vi "mdps.vi"() -> ()   [LabVIEW 2015]
uses:
  <vilib>/Utility/error.llb/DialogType.ctl
  <vilib>/DAQmx/read.llb/DAQmx Read (Digital Bool 1Line 1Point).vi
  <vilib>/DAQmx/read.llb/DAQmx Read (Analog 1D DBL NChan 1Samp).vi
  <vilib>/DAQmx/write.llb/DAQmx Write (Analog 1D DBL NChan 1Samp).vi
  <vilib>/DAQmx/write.llb/DAQmx Write (Digital Bool 1Line 1Point).vi
  <vilib>/DAQmx/write.llb/DAQmx Write (Counter Frequency 1Chan 1Samp).vi
  <vilib>/DAQmx/create/channels.llb/DAQmx Create Channel (CO-Pulse Generation-Frequency).vi
  <vilib>/DAQmx/configure/timing.llb/DAQmx Timing (Implicit).vi
  mdps_global.vi
  <vilib>/DAQmx/miscellaneous.llb/DAQmx Fill In Error Info.vi
  <vilib>/DAQmx/create/channels.llb/DAQmx Create Channel (AI-Voltage-Basic).vi
  <vilib>/DAQmx/create/channels.llb/DAQmx Create Channel (DI-Digital Input).vi
  <vilib>/DAQmx/create/channels.llb/DAQmx Create Channel (AO-Voltage-Basic).vi
  <vilib>/DAQmx/create/channels.llb/DAQmx Create Channel (DO-Digital Output).vi
  <vilib>/Utility/inputDevices.llb/mouseAcquire.vi
  <vilib>/Utility/inputDevices.llb/closeMouse.vi
  <vilib>/DAQmx/configure/timing.llb/DAQmx Timing (Sample Clock).vi
  <vilib>/DAQmx/read.llb/DAQmx Read (Analog 2D DBL NChan NSamp).vi
  <vilib>/Instr/_visa.llb/VISA Configure Serial Port (Instr).vi
panel:
  out "read buffer":string
  in  "vel":i32 min=0 max=1000 step=20
  out "count 3":i32
  out "solinit":bool
  out "count 2":i32
  out "manual":bool
  out "Waveform Chart 2":dynamicdata(graph)
  out "lastval":dbl[](array[numeric])
  out "count":i32
  in  "steering":dbl(knob) min=-0.45 max=0.45 step=0.005 scale=-0.45..0.45
  out "Waveform Chart":dynamicdata(graph)
  out "coerced(x)":dbl[](array[numeric])
  out "data 2":bool
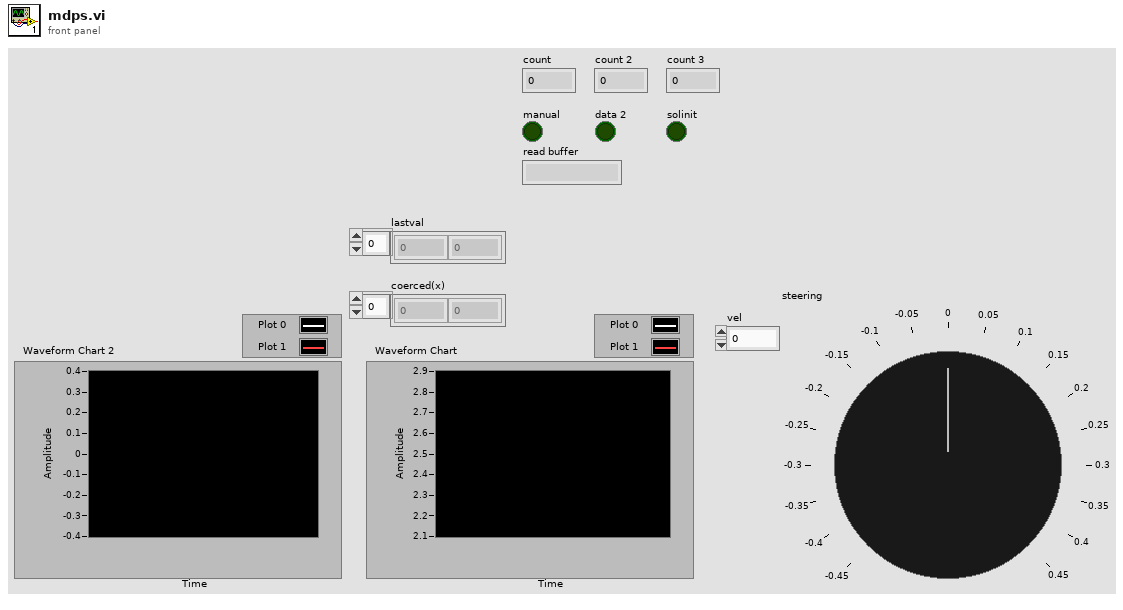
[diagram p1: front panel]
types:
  T1 = typedef "DialogType.ctl" = u16
  T2 = cluster{"button 1":bool, "button 2":bool, "button 3":bool, "button 4":bool}
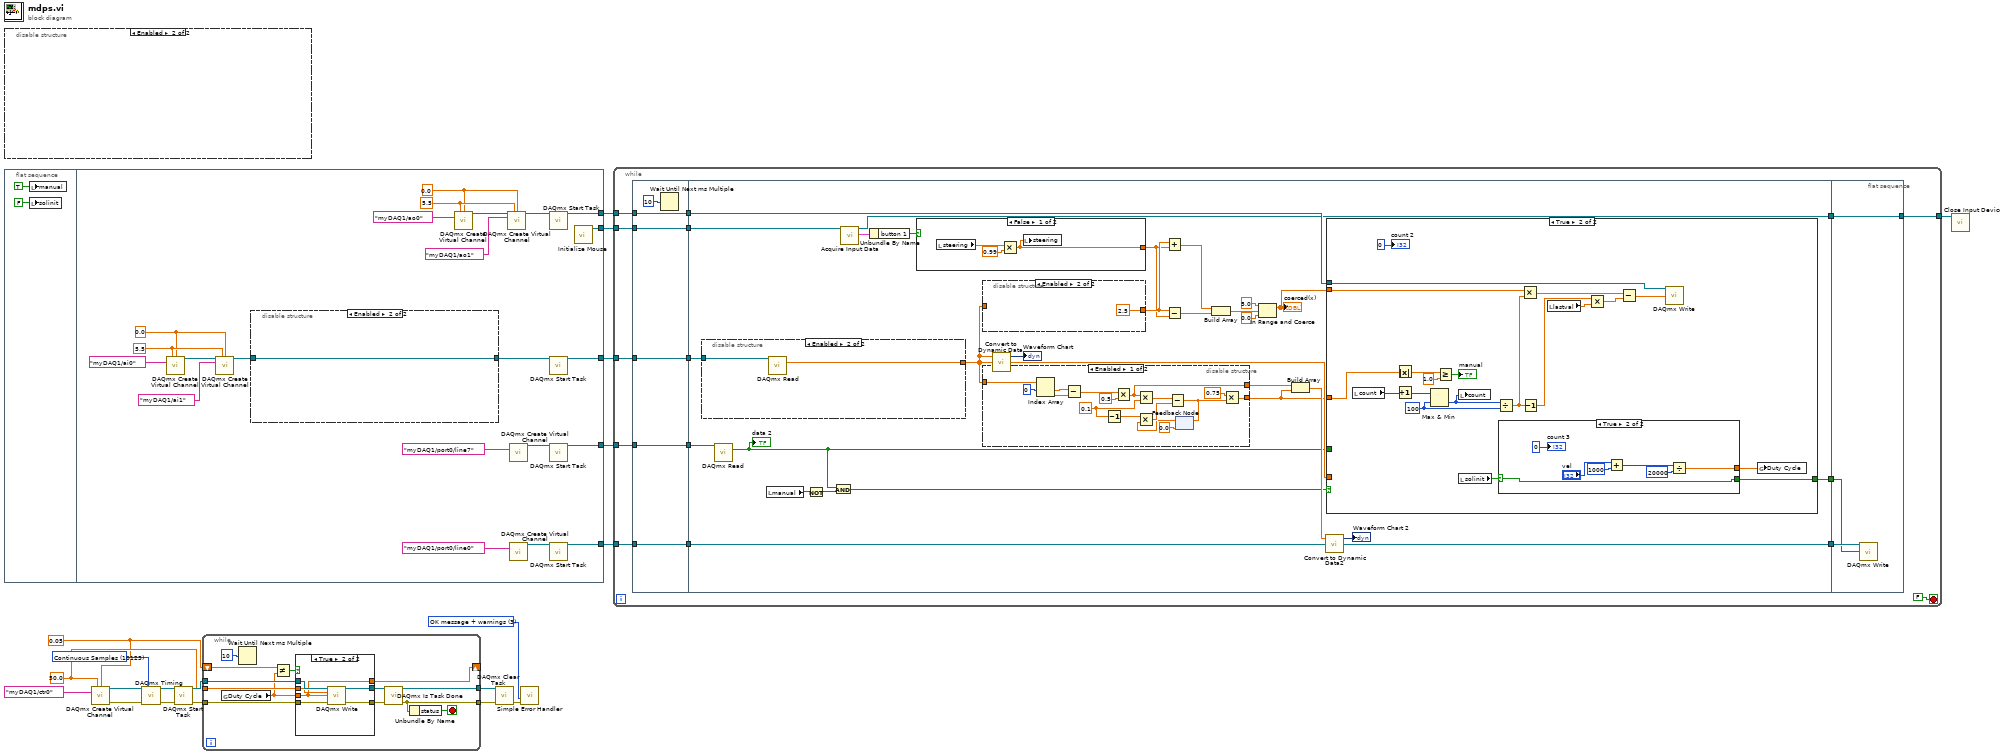
[diagram p0: block diagram]
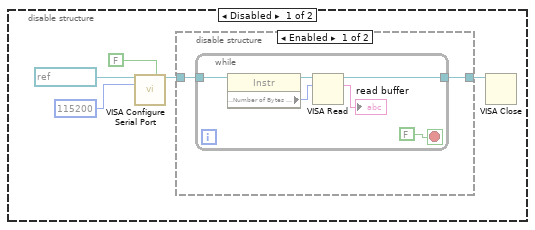
[diagram p2: hidden frame]
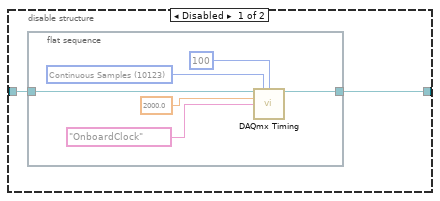
[diagram p5: hidden frame]
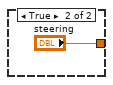
[diagram p6: hidden frame]
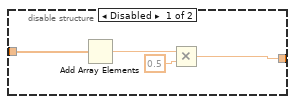
[diagram p7: hidden frame]
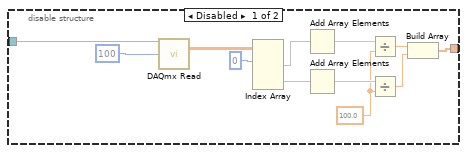
[diagram p8: hidden frame]
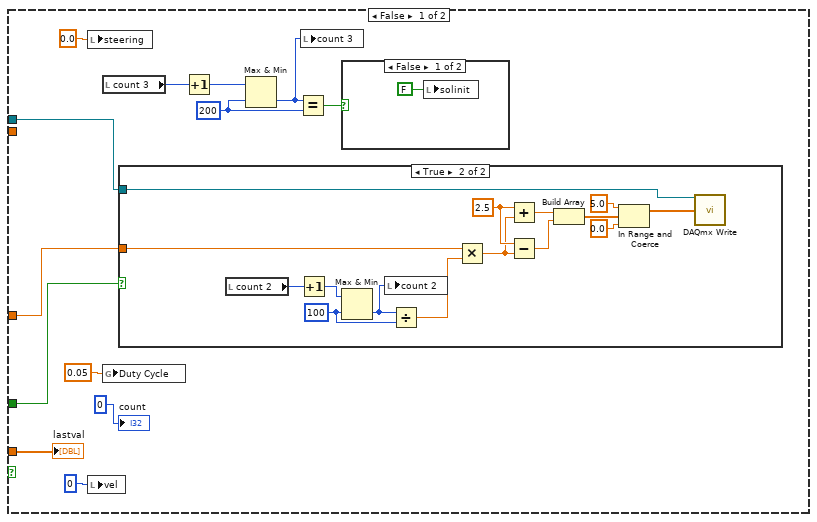
[diagram p10: hidden frame]
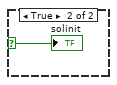
[diagram p11: hidden frame]
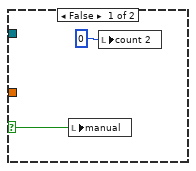
[diagram p12: hidden frame]
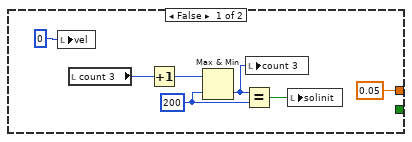
[diagram p13: hidden frame]
diagram:
  w4 = 0.05 ("Duty Cycle")
  w5 = 50.0 ("Frequency")
  w6 = T1 3 items=["no dialog", "OK message", "continue or stop message", "OK message + warnings", "continue/stop + warnings"] ("type of dialog (OK msg:1)")
  w9 = 10123 items=["Finite Samples"=10178, "Continuous Samples"=10123] ("sample mode")
  n1 = disable-structure shown="Enabled" {
    frame Disabled {
      n2 = call-poly "VISA Configure Serial Port"("VISA resource name"=refnum<visa-resource-name> "COM8", "Enable Termination\nChar (T)"=FALSE ("Enable Termination\nChar (T)"), "baud rate (9600)"=u32 115200) -> ("VISA resource name out"=w23:refnum<visa-resource-name>)  [unwired: 6 in, 6 out]
      n3 = disable-structure shown="Enabled" {
        disable-tunnel: w23 -> [w27 w34]
        disable-tunnel: [w26 w34] -> w22
        frame Enabled {
          n4 = while {
            tunnel: w27 -> [w31]
            tunnel: [w32] -> w26
            stop <- FALSE stop-if-true
            n5 = property class="Instr"(reference=w31) -> (reference out=w30:refnum<visa-resource-name>, "Serial Settings:Number of Bytes at Serial Port"=w29:u32)  [unwired: 1 in, 1 out]
            n6 = VISA Read(VISA resource name=w30, byte count=w29) -> (VISA resource name out=w32:refnum<visa-resource-name>, read buffer=→"read buffer":string)  [unwired: 1 in, 2 out]
          }
        }
        frame Disabled {
        }
      }
      n7 = VISA Close(VISA resource name=w22) -> ()  [unwired: 1 in, 1 out]
    }
    frame Enabled {
    }
  }
  n8 = flat-sequence {
    tunnel: [w53] -> w20
    tunnel: [w50] -> w19
    tunnel: [w46] -> w18
    tunnel: [w38] -> w3
    tunnel: [w37] -> w2
    frame #0 {
      n9 = local write "manual"(TRUE) -> ()
      n10 = local write "solinit"(FALSE) -> ()
    }
    frame #1 {
      w44 = 0.0 ("minimum value")
      w45 = 5.5 ("maximum value")
      w54 = 0.0 ("minimum value")
      w55 = 5.5 ("maximum value")
      n11 = call-poly <vilib>:"DAQmx Create Virtual Channel.vi"("maximum value"=w55, "minimum value"=w54, "physical channels"=tag "myDAQ1/ai0" ("Physical Channel")) -> ("task out"=w57:refnum<k21>)  [unwired: 11 in, 1 out]
      n12 = call-poly <vilib>:"DAQmx Create Virtual Channel.vi"("task in"=w57, "maximum value"=w55, "minimum value"=w54, "physical channels"=tag "myDAQ1/ai1") -> ("task out"=w43:refnum<k21>)  [unwired: 10 in, 1 out]
      n13 = disable-structure shown="Enabled" {
        disable-tunnel: w43 -> [w60 w67]
        disable-tunnel: [w59 w67] -> w42
        frame Disabled {
          n14 = flat-sequence {
            tunnel: w60 -> [w66]
            tunnel: [w65] -> w59
            frame #0 {
              w61 = 10123 items=["Finite Samples"=10178, "Continuous Samples"=10123, "Hardware Timed Single Point"=12522] ("sample mode")
              n15 = call-poly <vilib>:"DAQmx Timing.vi"("task/channels in"=w66, "sample mode"=w61, "samples per channel"=100, "rate"=2000.0, "source"=tag "OnboardClock") -> ("task out"=w65:refnum<k21>)  [unwired: 9 in, 1 out]
            }
          }
        }
        frame Enabled {
        }
      }
      n16 = call-poly <vilib>:"DAQmx Create Virtual Channel.vi"("maximum value"=w45, "minimum value"=w44, "physical channels"=tag "myDAQ1/ao0") -> ("task out"=w48:refnum<k21>)  [unwired: 11 in, 1 out]
      n17 = call-poly <vilib>:"DAQmx Create Virtual Channel.vi"("task in"=w48, "maximum value"=w45, "minimum value"=w44, "physical channels"=tag "myDAQ1/ao1") -> ("task out"=w41:refnum<k21>)  [unwired: 10 in, 1 out]
      n18 = call-poly <vilib>:"DAQmx Create Virtual Channel.vi"("lines"=tag "myDAQ1/port0/line7") -> ("task out"=w51:refnum<k21>)  [unwired: 13 in, 1 out]
      n19 = call-poly <vilib>:"DAQmx Create Virtual Channel.vi"("lines"=tag "myDAQ1/port0/line0") -> ("task out"=w40:refnum<k21>)  [unwired: 13 in, 1 out]
      n20 = call <vilib>:"DAQmx Start Task.vi"("task/channels in"=w41) -> ("task out"=w46:refnum<k21>)  [unwired: 13 in, 1 out]
      n21 = call <vilib>:"DAQmx Start Task.vi"("task/channels in"=w42) -> ("task out"=w53:refnum<k21>)  [unwired: 13 in, 1 out]
      n22 = call <vilib>:"DAQmx Start Task.vi"("task/channels in"=w51) -> ("task out"=w50:refnum<k21>)  [unwired: 13 in, 1 out]
      n23 = call <vilib>:"DAQmx Start Task.vi"("task/channels in"=w40) -> ("task out"=w38:refnum<k21>)  [unwired: 13 in, 1 out]
      n24 = call <vilib>:"Initialize Mouse.vi"() -> ("device ID"=w37:refnum<k1>)  [unwired: 10 in, 1 out]
    }
  }
  n25 = call-poly <vilib>:"DAQmx Create Virtual Channel.vi"("frequency"=w5, "duty cycle"=w4, "counter"=tag "myDAQ1/ctr0" ("Counter(s)")) -> ("task out"=w14:refnum<k21>, "error out"=w17:errorcluster)  [unwired: 11 in]
  n26 = call-poly <vilib>:"DAQmx Timing.vi"("task/channels in"=w14, "sample mode"=w9, "error in"=w17) -> ("task out"=w10:refnum<k21>, "error out"=w11:errorcluster)  [unwired: 11 in]
  n27 = call <vilib>:"DAQmx Start Task.vi"("task/channels in"=w10, "error in"=w11) -> ("task out"=w13:refnum<k21>, "error out"=w16:errorcluster)  [unwired: 12 in]
  n28 = while {
    tunnel: w16 -> [w75]
    tunnel: w13 -> [w76]
    tunnel: [w80] -> w12
    tunnel: [w79] -> w7
    tunnel: w5 -> [w74]
    shift-right: [w71] -> _
    shift-left: w4 -> [w72]
    stop <- w69 stop-if-true
    n29 = global read "mdps_global.vi" "Duty Cycle"() -> (w68:dbl)
    n30 = Wait Until Next ms Multiple(millisecond multiple=u32 10) -> ()  [unwired: 1 out]
    n31 = Not Equal?(x=w72, y=w68) -> (x != y?=w73:bool)
    n32 = case shown="True" w73 {
      tunnel: [w83 w89] -> w78
      tunnel: [w82 w88] -> w77
      tunnel: w76 -> [w83 w87]
      tunnel: w75 -> [w82 w86]
      tunnel: w74 -> [_ w85]
      tunnel: w68 -> [w81 w84]
      tunnel: [w81 w84] -> w71
      frame False {
      }
      frame True {
        n33 = call-poly <vilib>:"DAQmx Write.vi"("task/channels in"=w87, "frequency"=w85, "duty cycle"=w84, "error in"=w86) -> ("task out"=w89:refnum<k21>, "error out"=w88:errorcluster)  [unwired: 9 in, 1 out]
      }
    }
    n34 = call <vilib>:"DAQmx Is Task Done.vi"("task/channels in"=w78, "error in"=w77) -> ("task out"=w80:refnum<k21>, "error out"=w79:errorcluster)  [unwired: 11 in, 1 out]
    n35 = Unbundle By Name(w79) -> ("status"=w69:bool)
  }
  n36 = call <vilib>:"DAQmx Clear Task.vi"("task in"=w12, "error in"=w7) -> ("error out"=w15:errorcluster)  [unwired: 13 in]
  n37 = call <vilib>:"Simple Error Handler.vi"("type of dialog (OK msg:1)"=w6, "error in (no error)"=w15) -> ()  [unwired: 3 in, 5 out]
  n38 = while {
    tunnel: w20 -> [w103]
    tunnel: w19 -> [w102]
    tunnel: w18 -> [w101]
    tunnel: w3 -> [w96]
    tunnel: w2 -> [w92]
    tunnel: [w90] -> w1
    stop <- FALSE stop-if-true
    n39 = flat-sequence {
      tunnel: w101 -> [w108]
      tunnel: w102 -> [w109]
      tunnel: w103 -> [w110]
      tunnel: [w110] -> w100
      tunnel: [w109] -> w99
      tunnel: [w108] -> w98
      tunnel: w96 -> [w106]
      tunnel: [w106] -> w95
      tunnel: [w105] -> w93
      tunnel: w92 -> [w105]
      tunnel: w100 -> [w126]
      tunnel: w99 -> [w137]
      tunnel: w98 -> [w136]
      tunnel: [w116] -> w97
      tunnel: w95 -> [w115]
      tunnel: [w115] -> w94
      tunnel: w93 -> [w114]
      tunnel: [w111] -> w91
      tunnel: w97 -> [w244]
      tunnel: w94 -> [w245]
      tunnel: w91 -> [w243]
      tunnel: [w243] -> w90
      frame #0 {
        n40 = Wait Until Next ms Multiple(millisecond multiple=u32 10) -> ()  [unwired: 1 out]
      }
      frame #1 {
        n41 = disable-structure shown="Enabled" {
          disable-tunnel: [w151 w159] -> w127
          disable-tunnel: w126 -> [w149 w160]
          frame Disabled {
            w154 = 100.0 ("y")
            n42 = call-poly <vilib>:"DAQmx Read.vi"("task/channels in"=w149, "number of samples per channel"=100) -> ("data"=w148:dbl[][])  [unwired: 11 in, 2 out]
            n43 = Index Array(array=w148, index (row) #1=0 ("disabled index (col)")) -> (element #1=w158:dbl[], element #2=w157:dbl[])  [unwired: 3 in]
            n44 = Add Array Elements(numeric array=w158) -> (sum=w156:dbl)
            n45 = Add Array Elements(numeric array=w157) -> (sum=w155:dbl)
            n46 = Divide(x=w156, y=w154) -> (x/y=w153:dbl)
            n47 = Divide(x=w155, y=w154) -> (x/y=w152:dbl)
            n48 = Build Array(w153, w152) -> (w151:dbl[])
          }
          frame Enabled {
            n49 = call-poly <vilib>:"DAQmx Read.vi"("task/channels in"=w160) -> ("data"=w159:dbl[])  [unwired: 12 in, 2 out]
          }
        }
        n50 = call-poly <vilib>:"DAQmx Read.vi"("task/channels in"=w137) -> ("data"=w117:bool)  [unwired: 12 in, 2 out]
        "data 2" <- w117
        n51 = local read "manual"() -> (w120:bool)
        n52 = Not(x=w120) -> (.not. x?=w119:bool)
        n53 = And(x=w117, y=w119) -> (x .and. y?=w118:bool)
        n54 = call-poly <vilib>:"Acquire Input Data.vi"("device ID"=w114) -> ("device ID"=w111:refnum<k1>, "button info"=w112:T2)  [unwired: 15 in, 2 out]
        n55 = Unbundle By Name(w112) -> ("button 1"=w113:bool)
        n56 = case shown="False" w113 {
          tunnel: [w138 "steering"] -> w122
          frame False {
            n57 = local read "steering"() -> (w139:dbl)
            n58 = Multiply(x=w139, y=0.99) -> (x*y=w138:dbl)
            n59 = local write "steering"(w138) -> ()
          }
          frame True {
          }
        }
        n60 = disable-structure shown="Enabled" {
          disable-tunnel: [w143 2.5] -> w132
          disable-tunnel: w127 -> [w142 _]
          frame Disabled {
            n61 = Add Array Elements(numeric array=w142) -> (sum=w145:dbl)
            n62 = Multiply(x=w145, y=0.5) -> (x*y=w143:dbl)
          }
          frame Enabled {
          }
        }
        n63 = disable-structure shown="Enabled" {
          disable-tunnel: [w173 _] -> w121
          disable-tunnel: w127 -> [w170 _]
          disable-tunnel: [w161 _] -> w123
          frame Enabled {
            w168 = 0.1 ("y")
            n64 = Index Array(array=w170, index #1=0 ("index")) -> (element #1=w172:dbl, element #2=w171:dbl)  [unwired: 1 in]
            n65 = Subtract(x=w172, y=w171) -> (x-y=w175:dbl)
            n66 = Decrement(x=w168) -> (x-1=w167:dbl)
            n67 = Multiply(x=w175, y=0.5) -> (x*y=w161:dbl)
            n68 = Multiply(x=w161, y=w168) -> (x*y=w166:dbl)
            n69 = feedback #1(0.0) -> (w163:dbl)
            n70 = Multiply(x=w167, y=w163) -> (x*y=w165:dbl)
            n71 = Subtract(x=w166, y=w165) -> (x-y=w164:dbl)
            n72 = feedback-in #1(w164) -> ()
            n73 = Multiply(x=0.75 ("gain"), y=w164) -> (x*y=w173:dbl)
          }
          frame Disabled {
          }
        }
        n74 = call "Convert to Dynamic Data"("Array"=w127) -> ("Dynamic Data Type"=→"Waveform Chart":dynamicdata)  [unwired: 3 in]
        n75 = Add(x=w132, y=w122) -> (x+y=w131:dbl)
        n76 = Subtract(x=w132, y=w122) -> (x-y=w130:dbl)
        n77 = Build Array(w131, w130) -> (w129:dbl[])
        n78 = In Range and Coerce(upper limit=5.0 ("maximum value"), x=w129, lower limit=0.0 ("minimum value")) -> (coerced(x)=w133:dbl[])  [unwired: 1 out]
        "coerced(x)" <- w133
        n79 = Build Array(w123, w121) -> (w125:dbl[])
        n80 = call "Convert to Dynamic Data2"("Array"=w125) -> ("Dynamic Data Type"=→"Waveform Chart 2":dynamicdata)  [unwired: 3 in]
        n81 = case shown="True" w118 {
          tunnel: w136 -> [w186 w228]
          tunnel: w133 -> [_ w219]
          tunnel: w127 -> [w188 _]
          tunnel: w121 -> [w185 w215]
          tunnel: w117 -> [w187 _]
          tunnel: [_ w209] -> w116
          frame False {
            w181 = 200 ("y")
            n82 = local write "steering"(0.0 ("steering")) -> ()
            n83 = local write "vel"(0 ("vel")) -> ()
            n84 = local read "count 3"() -> (w182:i32)
            n85 = global write "mdps_global.vi" "Duty Cycle"(0.05 ("Duty Cycle")) -> ()
            n86 = case shown="True" w187 {
              selector: w187 -> [w193 _]
              tunnel: w186 -> [_ w208]
              tunnel: w185 -> [_ w196]
              frame False {
                n87 = local write "manual"(w193) -> ()
                n88 = local write "count 2"(0 ("count 2")) -> ()
              }
              frame True {
                w197 = 100 ("y")
                w205 = 2.5
                n89 = local read "count 2"() -> (w200:i32)
                n90 = Increment(x=w200) -> (x+1=w199:i32)
                n91 = Max & Min(x=w199, y=w197) -> (min(x,y)=w198:i32)  [unwired: 1 out]
                n92 = local write "count 2"(w198) -> ()
                n93 = Divide(x=w198, y=w197) -> (x/y=w194:dbl)
                n94 = Multiply(x=w196, y=w194) -> (x*y=w195:dbl)
                n95 = Add(x=w205, y=w195) -> (x+y=w206:dbl)
                n96 = Subtract(x=w205, y=w195) -> (x-y=w207:dbl)
                n97 = Build Array(w206, w207) -> (w202:dbl[])
                n98 = In Range and Coerce(upper limit=5.0 ("maximum value"), x=w202, lower limit=0.0 ("minimum value")) -> (coerced(x)=w201:dbl[])  [unwired: 1 out]
                n99 = call-poly <vilib>:"DAQmx Write.vi"("task/channels in"=w208, "data"=w201) -> ()  [unwired: 11 in, 3 out]
              }
            }
            n100 = Increment(x=w182) -> (x+1=w183:i32)
            n101 = Max & Min(x=w183, y=w181) -> (min(x,y)=w179:i32)  [unwired: 1 out]
            n102 = Equal?(x=w179, y=w181) -> (x = y?=w180:bool)
            n103 = local write "count 3"(w179) -> ()
            n104 = case shown="False" w180 {
              selector: w180 -> [_ w191]
              frame False {
                n105 = local write "solinit"(FALSE ("solinit")) -> ()
              }
              frame True {
                "solinit" <- w191
              }
            }
            "count" <- 0
            "lastval" <- w188
          }
          frame True {
            w225 = 100 ("y")
            n106 = local read "count"() -> (w227:i32)
            n107 = Absolute Value(x=w215) -> (abs(x)=w216:dbl)
            n108 = Increment(x=w227) -> (x+1=w226:i32)
            n109 = Max & Min(x=w226, y=w225) -> (min(x,y)=w224:i32)  [unwired: 1 out]
            n110 = Greater Or Equal?(x=w216, y=1.0) -> (x >= y?=→"manual":bool)
            n111 = local write "count"(w224) -> ()
            n112 = local read "solinit"() -> (w211:bool)
            n113 = Divide(x=w224, y=w225) -> (x/y=w220:dbl)
            n114 = case shown="True" w211 {
              selector: w211 -> [_ w236]
              tunnel: [0.05 ("Duty Cycle") w238] -> w210
              tunnel: [_ w236] -> w209
              frame False {
                w233 = 200 ("y")
                n115 = local write "vel"(0 ("vel")) -> ()
                n116 = local read "count 3"() -> (w234:i32)
                n117 = Increment(x=w234) -> (x+1=w235:i32)
                n118 = Max & Min(x=w235, y=w233) -> (min(x,y)=w232:i32)  [unwired: 1 out]
                n119 = Equal?(x=w232, y=w233) -> (x = y?=w231:bool)
                n120 = local write "count 3"(w232) -> ()
                n121 = local write "solinit"(w231) -> ()
              }
              frame True {
                n122 = Add(x="vel", y=1000) -> (x+y=w239:i32)
                n123 = Divide(x=w239, y=20000) -> (x/y=w238:dbl)
                "count 3" <- 0 ("count 3")
              }
            }
            n124 = Multiply(x=w219, y=w220) -> (x*y=w217:dbl[])
            n125 = Decrement(x=w220) -> (x-1=w223:dbl)
            n126 = local read "lastval"() -> (w222:dbl[])
            n127 = Multiply(x=w223, y=w222) -> (x*y=w221:dbl[])
            n128 = Subtract(x=w217, y=w221) -> (x-y=w218:dbl[])
            n129 = call-poly <vilib>:"DAQmx Write.vi"("task/channels in"=w228, "data"=w218) -> ()  [unwired: 11 in, 3 out]
            n130 = global write "mdps_global.vi" "Duty Cycle"(w210) -> ()
            "count 2" <- 0
          }
        }
      }
      frame #2 {
        n131 = call-poly <vilib>:"DAQmx Write.vi"("task/channels in"=w245, "data"=w244) -> ()  [unwired: 11 in, 3 out]
      }
    }
  }
  n132 = call-poly <vilib>:"Close Input Device.vi"("device ID"=w1) -> ()  [unwired: 9 in, 1 out]
